vi "Set Range.vi"(0 "object in":refnum<class "HPS-17000-PowerModule.lvclass">, 5 "Range":T1, 11 "Error In":errorcluster) -> (4 "object out":refnum<class "HPS-17000-PowerModule.lvclass">, 15 "Error Out":errorcluster)   [LabVIEW 2023, in "HPS-17000-PowerModule.lvlib" / "HPS-17000-PowerModule.lvclass"]
uses:
  HPS-17000-PowerModule.lvclass
  builds/PowerModuleInterface/PowerModuleInterface.lvlibp/Classes/PowerModule_interface/Range.ctl
  <instrlib>/HPS-17000/Client Facing Datatypes/Range.ctl
  <instrlib>/HPS-17000/Internal/Set Mode Multi.vi
  <instrlib>/HPS-17000/HPS-17000.lvclass
  builds/PowerModuleInterface/PowerModuleInterface.lvlibp/Classes/PowerModule_interface/PowerModuleInterface.lvclass
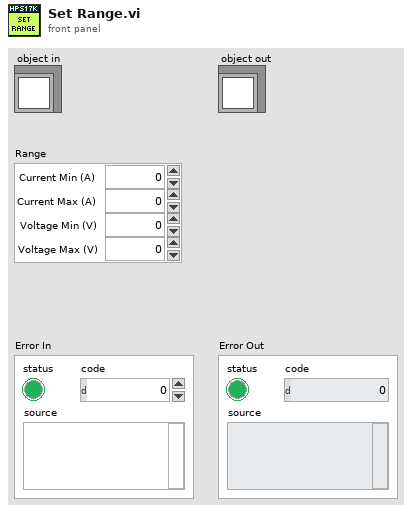
[diagram p1: front panel]
types:
  T1 = typedef "PowerModuleInterface.lvlibp/PowerModuleInterface.lvclass/Range.ctl" = cluster{"Current Max (A)":dbl, "Current Min (A)":dbl, "Voltage Max (V)":dbl, "Voltage Min (V)":dbl}
  T2 = typedef "HPS-17000-PowerModule.lvlib/HPS-17000-PowerModule.lvclass/ObjectAttributes.ctl" = cluster{"JSON Config Path":path, "Configuration":T3, "GM ID":string, "HPS17000 Refs":refnum<class "HPS-17000.lvclass">[], "connected":bool, "reserved":bool, "events":T5, "nibatterycycler_grpc_Setpoint":T6, "last timestamp":i64, "mode":T7, "range":T1, "measurement array":T8[]}
  T3 = typedef "HPS-17000-PowerModule.lvlib/HPS-17000-PowerModule.lvclass/Configuration.ctl" = cluster{"TSN NIC IP Address":string, "HPS17000 IP Addresses":string[], "HPS Topology":enum16{"SINGLE", "MULTI"}, "Setpoint Stream Config":T4, "Measurement Array Size":i32}
  T4 = typedef "Cycler.lvclass/Setpoint Stream Basic Config.ctl" = cluster{"local address":string, "receiver port":u16}
  T5 = typedef "HPS-17000.lvclass/Multi-Cycler Events.ctl" = cluster{"heartbeats events":refnum<user-event>[], "faults events":refnum<user-event>[], "network sync event":refnum<user-event>[], "setpoint status event":refnum<user-event>[]}
  T6 = typedef "NI_BC_client.lvlib/nibatterycycler_grpc_Setpoint.ctl" = cluster{"voltage":sgl, "current":sgl, "min_power":sgl, "max_power":sgl, "resistance":sgl}
  T7 = typedef "HPS-17000-PowerModule.lvlib/HPS-17000-PowerModule.lvclass/Mode.ctl" = u16
  T8 = typedef "PowerModuleInterface.lvlibp/PowerModuleInterface.lvclass/Measurements.ctl" = cluster{"measured voltage (V)":dbl, "measured current (A)":dbl, "setpoint voltage (V)":dbl, "setpoint current (A)":dbl, "timestamp":dbl}
  T9 = typedef "HPS-17000.lvclass/Range.ctl" = u8
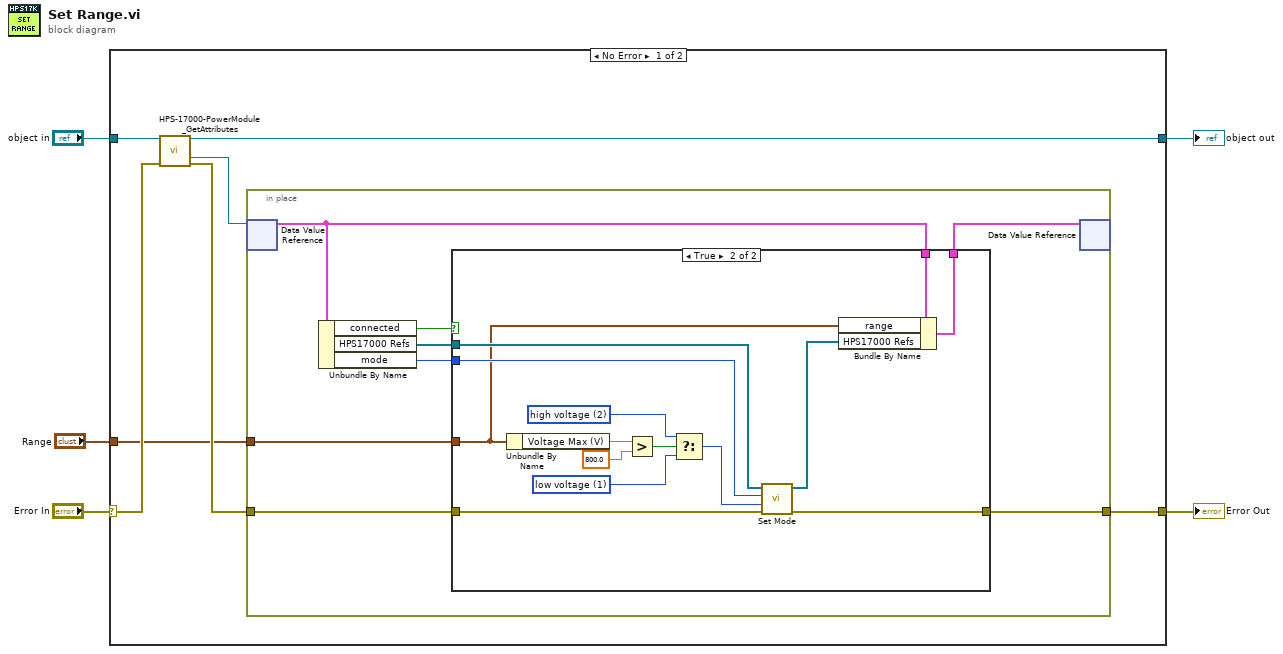
[diagram p0: block diagram]
diagram:
  n1 = case shown="No Error" "Error In" {
    selector: "Error In" -> [w12 w38]
    tunnel: [w8 w37] -> w3
    tunnel: [w9 w38] -> w2
    tunnel: "object in" -> [w7 w37]
    tunnel: "Range" -> [w6 _]
    frame No Error {
      n2 = call "HPS-17000-PowerModule_GetAttributes.vi"("reference in"=w7, "Error In"=w12) -> ("reference out"=w8:refnum<class "HPS-17000-PowerModule.lvclass">, "DataRef"=w11:refnum<data-value>, "Error Out"=w10:errorcluster)  [unwired: 10 in, 1 out]
      n3 = in-place {
        in-place-border: w10 -> [w13]
        in-place-border: [w18] -> w9
        in-place-border: w6 -> [w14]
        n4 = in-place-dvr #1(w11) -> (w19:T2)  [unwired: 1 out]
        n5 = Unbundle By Name(w19) -> ("connected"=w16:bool, "HPS17000 Refs"=w17:refnum<class "HPS-17000.lvclass">[], "mode"=w15:T7)
        n6 = case shown="True" w16 {
          tunnel: [w22 w36] -> w20
          tunnel: w19 -> [w22 w35]
          tunnel: w13 -> [w21 w34]
          tunnel: [w21 w31] -> w18
          tunnel: w17 -> [_ w33]
          tunnel: w15 -> [_ w30]
          tunnel: w14 -> [_ w29]
          frame False {
          }
          frame True {
            w25 = T9 2 items=["low voltage"=1, "high voltage"=2] ("range")
            w24 = T9 1 items=["low voltage"=1, "high voltage"=2] ("range")
            n7 = Unbundle By Name(w29) -> ("Voltage Max (V)"=w28:dbl)
            n8 = Greater?(x=w28, y=800.0) -> (0:w26:bool)
            n9 = Select(t=w25, s=w26, f=w24) -> (s? t:f=w23:T9)
            n10 = call-poly <instrlib>:"Set Mode.vi"("error in"=w34, "range"=w23, "mode"=w30, "cycler refs in"=w33) -> ("error out"=w31:errorcluster, "cycler refs out"=w32:refnum<class "HPS-17000.lvclass">[])  [unwired: 6 in]
            n11 = Bundle By Name(cluster=w35, "range"=w29, "HPS17000 Refs"=w32) -> (w36:T2)
          }
        }
        n12 = in-place-dvr #1(w20) -> ()  [unwired: 2 out]
      }
    }
    frame Error {
    }
  }
  "Error Out" <- w2
  "object out" <- w3
